vi "Create Serial Input Channel CSI-2 IO x4.vi"() -> (4 "serial input csi-2 io x4":T4)   [LabVIEW 2020, in "GettingStarted_Acq_Tap_148X_FPGA.lvlib"]
uses:
  GettingStarted_Acq_Tap_148X_FPGA.lvlib
  Types/Serial Input Channel IO.ctl
  Types/Serial Input Channel IO 32b.ctl
  Types/Serial Input Channel IO 64b.ctl
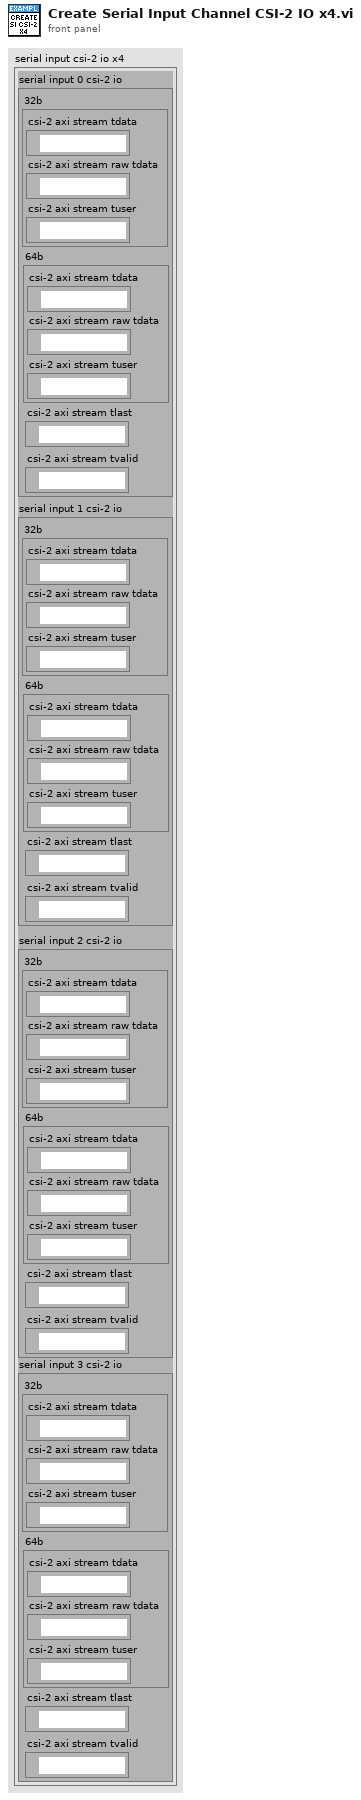
[diagram p1: front panel]
types:
  T1 = typedef "GettingStarted_Acq_Tap_148X_FPGA.lvlib/Serial Input Channel IO.ctl" = cluster{"32b":T2, "64b":T3, "csi-2 axi stream tlast":refnum<k21>, "csi-2 axi stream tvalid":refnum<k21>}
  T2 = typedef "GettingStarted_Acq_Tap_148X_FPGA.lvlib/Serial Input Channel IO 32b.ctl" = cluster{"csi-2 axi stream tdata":refnum<k21>, "csi-2 axi stream raw tdata":refnum<k21>, "csi-2 axi stream tuser":refnum<k21>}
  T3 = typedef "GettingStarted_Acq_Tap_148X_FPGA.lvlib/Serial Input Channel IO 64b.ctl" = cluster{"csi-2 axi stream tdata":refnum<k21>, "csi-2 axi stream raw tdata":refnum<k21>, "csi-2 axi stream tuser":refnum<k21>}
  T4 = cluster{"serial input 0 csi-2 io":T1, "serial input 1 csi-2 io":T1, "serial input 2 csi-2 io":T1, "serial input 3 csi-2 io":T1}
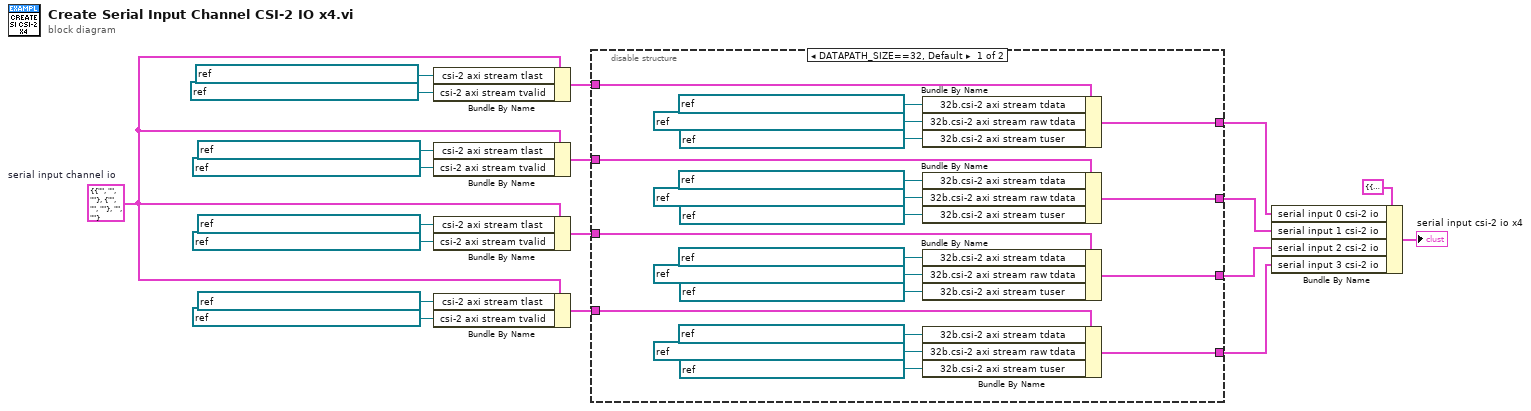
[diagram p0: block diagram]
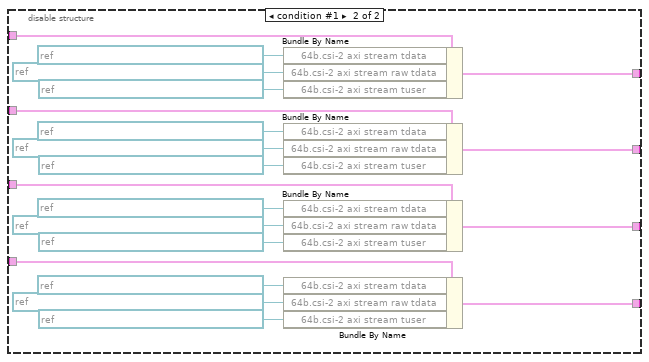
[diagram p2: hidden frame]
diagram:
  w17 = T1 {"32b"={"csi-2 axi stream tdata"="", "csi-2 axi stream raw tdata"="", "csi-2 axi stream tuser"=""}, "64b"={"csi-2 axi stream tdata"="", "csi-2 axi stream raw tdata"="", "csi-2 axi stream tuser"=""}, "csi-2 axi stream tlast"="", "csi-2 axi stream tvalid"=""}  # serial input channel io
  n1 = Bundle By Name(cluster=w17, "csi-2 axi stream tlast"=refnum<k21> "IO Socket\\SI 0 CSI-2 AXI Stream TLast" ("FPGA I/O In"), "csi-2 axi stream tvalid"=refnum<k21> "IO Socket\\SI 0 CSI-2 AXI Stream TValid" ("FPGA I/O In")) -> (w8:T1)
  n2 = Bundle By Name(cluster=w17, "csi-2 axi stream tlast"=refnum<k21> "IO Socket\\SI 1 CSI-2 AXI Stream TLast" ("FPGA I/O In"), "csi-2 axi stream tvalid"=refnum<k21> "IO Socket\\SI 1 CSI-2 AXI Stream TValid" ("FPGA I/O In")) -> (w7:T1)
  n3 = Bundle By Name(cluster=w17, "csi-2 axi stream tlast"=refnum<k21> "IO Socket\\SI 2 CSI-2 AXI Stream TLast" ("FPGA I/O In"), "csi-2 axi stream tvalid"=refnum<k21> "IO Socket\\SI 2 CSI-2 AXI Stream TValid" ("FPGA I/O In")) -> (w6:T1)
  n4 = Bundle By Name(cluster=w17, "csi-2 axi stream tlast"=refnum<k21> "IO Socket\\SI 3 CSI-2 AXI Stream TLast" ("FPGA I/O In"), "csi-2 axi stream tvalid"=refnum<k21> "IO Socket\\SI 3 CSI-2 AXI Stream TValid" ("FPGA I/O In")) -> (w5:T1)
  n5 = disable-structure shown="DATAPATH_SIZE==32, Default" {
    disable-tunnel: w8 -> [w39 w57]
    disable-tunnel: w7 -> [w38 w46]
    disable-tunnel: w6 -> [w37 w45]
    disable-tunnel: w5 -> [w36 w44]
    disable-tunnel: [w23 w43] -> w4
    disable-tunnel: [w22 w42] -> w3
    disable-tunnel: [w21 w41] -> w2
    disable-tunnel: [w20 w40] -> w1
    frame condition #0 (active) {
      n6 = Bundle By Name(cluster=w39, "32b.csi-2 axi stream tdata"=refnum<k21> "IO Socket\\SI 0 CSI-2 AXI Stream TData" ("FPGA I/O In"), "32b.csi-2 axi stream raw tdata"=refnum<k21> "IO Socket\\SI 0 CSI-2 AXI Stream Raw TData" ("FPGA I/O In"), "32b.csi-2 axi stream tuser"=refnum<k21> "IO Socket\\SI 0 CSI-2 AXI Stream TUser" ("FPGA I/O In")) -> (w23:T1)
      n7 = Bundle By Name(cluster=w38, "32b.csi-2 axi stream tdata"=refnum<k21> "IO Socket\\SI 1 CSI-2 AXI Stream TData" ("FPGA I/O In"), "32b.csi-2 axi stream raw tdata"=refnum<k21> "IO Socket\\SI 1 CSI-2 AXI Stream Raw TData" ("FPGA I/O In"), "32b.csi-2 axi stream tuser"=refnum<k21> "IO Socket\\SI 1 CSI-2 AXI Stream TUser" ("FPGA I/O In")) -> (w22:T1)
      n8 = Bundle By Name(cluster=w37, "32b.csi-2 axi stream tdata"=refnum<k21> "IO Socket\\SI 2 CSI-2 AXI Stream TData" ("FPGA I/O In"), "32b.csi-2 axi stream raw tdata"=refnum<k21> "IO Socket\\SI 2 CSI-2 AXI Stream Raw TData" ("FPGA I/O In"), "32b.csi-2 axi stream tuser"=refnum<k21> "IO Socket\\SI 2 CSI-2 AXI Stream TUser" ("FPGA I/O In")) -> (w21:T1)
      n9 = Bundle By Name(cluster=w36, "32b.csi-2 axi stream tdata"=refnum<k21> "IO Socket\\SI 3 CSI-2 AXI Stream TData" ("FPGA I/O In"), "32b.csi-2 axi stream raw tdata"=refnum<k21> "IO Socket\\SI 3 CSI-2 AXI Stream Raw TData" ("FPGA I/O In"), "32b.csi-2 axi stream tuser"=refnum<k21> "IO Socket\\SI 3 CSI-2 AXI Stream TUser" ("FPGA I/O In")) -> (w20:T1)
    }
    frame condition #1 {
      n10 = Bundle By Name(cluster=w57, "64b.csi-2 axi stream tdata"=refnum<k21> "IO Socket\\SI 0 CSI-2 AXI Stream TData" ("FPGA I/O In"), "64b.csi-2 axi stream raw tdata"=refnum<k21> "IO Socket\\SI 0 CSI-2 AXI Stream Raw TData" ("FPGA I/O In"), "64b.csi-2 axi stream tuser"=refnum<k21> "IO Socket\\SI 0 CSI-2 AXI Stream TUser" ("FPGA I/O In")) -> (w43:T1)
      n11 = Bundle By Name(cluster=w46, "64b.csi-2 axi stream tdata"=refnum<k21> "IO Socket\\SI 1 CSI-2 AXI Stream TData" ("FPGA I/O In"), "64b.csi-2 axi stream raw tdata"=refnum<k21> "IO Socket\\SI 1 CSI-2 AXI Stream Raw TData" ("FPGA I/O In"), "64b.csi-2 axi stream tuser"=refnum<k21> "IO Socket\\SI 1 CSI-2 AXI Stream TUser" ("FPGA I/O In")) -> (w42:T1)
      n12 = Bundle By Name(cluster=w45, "64b.csi-2 axi stream tdata"=refnum<k21> "IO Socket\\SI 2 CSI-2 AXI Stream TData" ("FPGA I/O In"), "64b.csi-2 axi stream raw tdata"=refnum<k21> "IO Socket\\SI 2 CSI-2 AXI Stream Raw TData" ("FPGA I/O In"), "64b.csi-2 axi stream tuser"=refnum<k21> "IO Socket\\SI 2 CSI-2 AXI Stream TUser" ("FPGA I/O In")) -> (w41:T1)
      n13 = Bundle By Name(cluster=w44, "64b.csi-2 axi stream tdata"=refnum<k21> "IO Socket\\SI 3 CSI-2 AXI Stream TData" ("FPGA I/O In"), "64b.csi-2 axi stream raw tdata"=refnum<k21> "IO Socket\\SI 3 CSI-2 AXI Stream Raw TData" ("FPGA I/O In"), "64b.csi-2 axi stream tuser"=refnum<k21> "IO Socket\\SI 3 CSI-2 AXI Stream TUser" ("FPGA I/O In")) -> (w40:T1)
    }
  }
  n14 = Bundle By Name(cluster=T4 {"serial input 0 csi-2 io"={"32b"={"csi-2 axi stream tdata"="", "csi-2 axi stream raw tdata"="", "csi-2 axi stream tuser"=""}, "64b"={"csi-2 axi stream tdata"="", "csi-2 axi stream raw tdata"="", "csi-2 axi stream tuser"=""}, "csi-2 axi stream tlast"="", "csi-2 axi stream tvalid"=""}, "serial input 1 csi-2 io"={"32b"={"csi-2 axi stream tdata"="", "csi-2 axi stream raw tdata"="", "csi-2 axi stream tuser"=""}, "64b"={"csi-2 axi stream tdata"="", "csi-2 axi stream raw tdata"="", "csi-2 axi stream tuser"=""}, "csi-2 axi stream tlast"="", "csi-2 axi stream tvalid"=""}, "serial input 2 csi-2 io"={"32b"={"csi-2 axi stream tdata"="", "csi-2 axi stream raw tdata"="", "csi-2 axi stream tuser"=""}, "64b"={"csi-2 axi stream tdata"="", "csi-2 axi stream raw tdata"="", "csi-2 axi stream tuser"=""}, "csi-2 axi stream tlast"="", "csi-2 axi stream tvalid"=""}, "serial input 3 csi-2 io"={"32b"={"csi-2 axi stream tdata"="", "csi-2 axi stream raw tdata"="", "csi-2 axi stream tuser"=""}, "64b"={"csi-2 axi stream tdata"="", "csi-2 axi stream raw tdata"="", "csi-2 axi stream tuser"=""}, "csi-2 axi stream tlast"="", "csi-2 axi stream tvalid"=""}}, "serial input 0 csi-2 io"=w4, "serial input 1 csi-2 io"=w3, "serial input 2 csi-2 io"=w2, "serial input 3 csi-2 io"=w1) -> (→"serial input csi-2 io x4":T4)
